vi "FTW-HTTPClient-GET.vi"(0 "HTTP Client":refnum<class "FTW-HTTPClient.lvclass">, 5 "Endpoint":string, 11 "error in":errorcluster) -> (4 "HTTP Client out":refnum<class "FTW-HTTPClient.lvclass">, 6 "Response Headers":string, 8 "Response Body":string, 15 "error out":errorcluster)   [LabVIEW 2012, in "FTW-HTTPClient.lvclass"]
uses:
  FTW-HTTPClient.lvclass
  FTW-HTTPClient.lvclass/FTW-HTTPClient.ctl
panel:
  # "Inputs"
  # "Outputs"
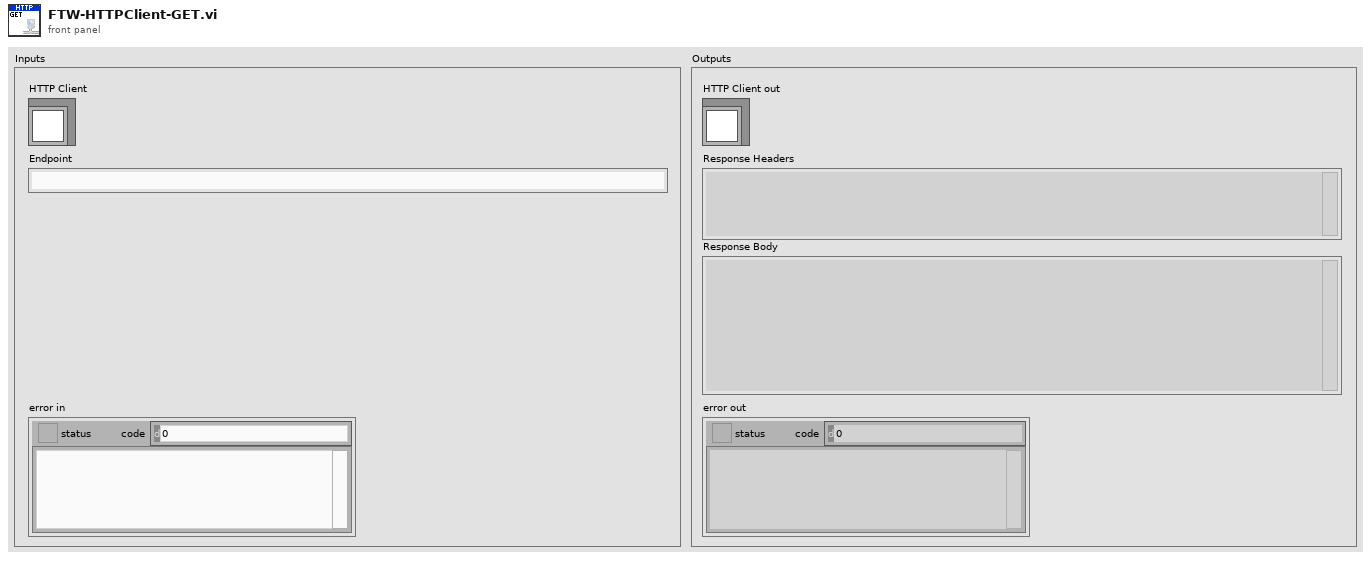
[diagram p1: front panel]
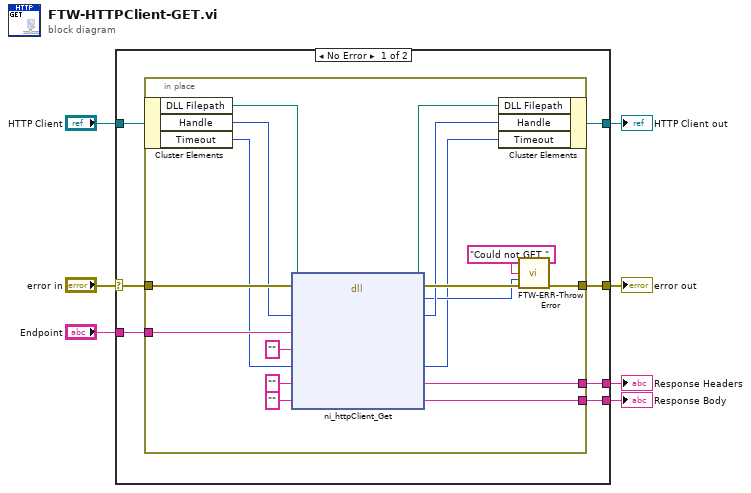
[diagram p0: block diagram]
diagram:
  n1 = case shown="No Error" "error in" {
    selector: "error in" -> [w13 w33]
    tunnel: "Endpoint" -> [w11 _]
    tunnel: [w10 w33] -> w6
    tunnel: "HTTP Client" -> [w14 w32]
    tunnel: [w12 w32] -> w5
    tunnel: [w9 _] -> w2
    tunnel: [w8 _] -> w1
    frame No Error {
      n2 = in-place {
        in-place-border: w13 -> [w27]
        in-place-border: w11 -> [w23]
        in-place-border: [w30] -> w10
        in-place-border: [w20] -> w9
        in-place-border: [w15] -> w8
        n3 = in-place-cluster #1(w14) -> ("DLL Filepath"=w29:path, "Handle"=w25:u32, "Timeout"=w16:i32)
        n4 = dll-call lib="ni_httpClient.*" fn="ni_httpClient_Get"(path in=w29, error in=w27, "Handle"=w25, "Endpoint"=w23, "Output Filepath"="", "Timeout"=w16, "Response Header"="", "Response Body"="") -> (path out=w28:path, error out=w26:errorcluster, "Return"=w18:i32, "Handle"=w19:u32, "Timeout"=w17:i32, "Response Header"=w20:string, "Response Body"=w15:string)  [unwired: 3 in]
        n5 = in-place-cluster #1("DLL Filepath"=w28, "Handle"=w19, "Timeout"=w17) -> (w12:refnum<class "FTW-HTTPClient.lvclass">)
        n6 = call "FTW-ERR-ThrowError.vi"("Error Message"="Could not GET.", "Error Code"=w18, "error in"=w26) -> ("error out"=w30:errorcluster)  [unwired: 12 in]
      }
    }
    frame Error {
    }
  }
  "error out" <- w6
  "HTTP Client out" <- w5
  "Response Headers" <- w2
  "Response Body" <- w1
